vi "create.vi"(8 "error in":errorcluster, 10 "type":string, 11 "Nominal Client":refnum<class "Nominal Client.lvclass">) -> (0 "error out":errorcluster, 3 "type":refnum<class "type.lvclass">)   [LabVIEW 2020, in "type.lvclass"]
uses:
  type.lvclass
  type.lvclass/type.ctl
  Nominal Client/Nominal Client.lvclass
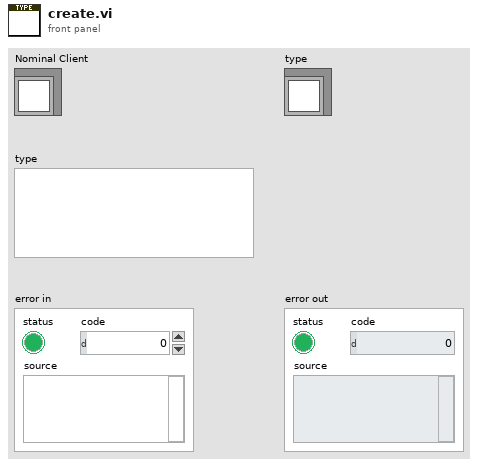
[diagram p1: front panel]
types:
  T1 = typedef "type.lvclass/typeData.ctl" = cluster{"rid":string, "name":string, "description":string, "propertyConfigs":T2, "createdAt":timestamp, "datasourceConfigs":T5[], "iconName":string}
  T2 = typedef "type.lvclass/properties.ctl" = T3[]
  T3 = typedef "type.lvclass/property.ctl" = cluster{"name":string, "value":T4}
  T4 = typedef "type.lvclass/property value.ctl" = cluster{"isRequired":bool, "description":string}
  T5 = typedef "type.lvclass/datasourceConfig.ctl" = cluster{"name":string, "v1":string[], "suggestedRefName":string}
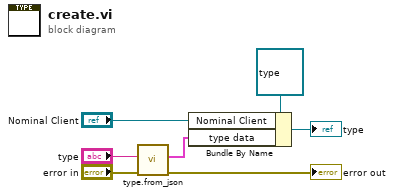
[diagram p0: block diagram]
diagram:
  n1 = call "type.from_json.vi"("error in"="error in", "json"="type") -> ("error out"=→"error out":errorcluster, "type data"=w5:T1)  [unwired: 8 in]
  n2 = Bundle By Name(cluster=refnum<class "type.lvclass"> refnum ("type"), "Nominal Client"="Nominal Client", "type data"=w5) -> (→"type":refnum<class "type.lvclass">)
